vi "AIT 1553 - Create RT Sysdef Tree Messages.vi"(7 "Called From SysDef API (F)":bool, 8 "error in":errorcluster, 9 "RT_Messages":T1[](array[typedef]), 10 "Section Ptr":T3 format="%.0x") -> (0 "error out":errorcluster)   [LabVIEW 2013, in "AIT 1553 Custom Device.lvlib"]
uses:
  AIT 1553 Custom Device.lvlib
  <vilib>/NI Veristand/Custom Device API/Custom Device Item Ref.ctl
  Controls/1553_RT_Message.ctl
  Controls/1553 Param.ctl
  <vilib>/NI Veristand/Custom Device API/Custom Device Channel Type.ctl
  <vilib>/NI Veristand/Custom Device API/Custom Device Channel.ctl
  Controls and Global/Global.vi
  <vilib>/NI Veristand/Custom Device API/Custom Device API.lvlib
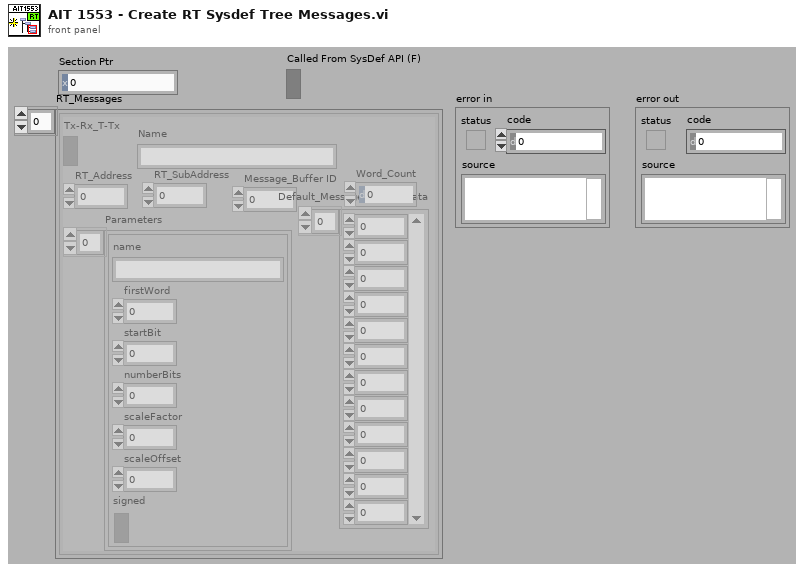
[diagram p1: front panel]
types:
  T1 = typedef "AIT 1553 Custom Device.lvlib/1553_RT_Message.ctl" = cluster{"RT_Address":u8, "RT_SubAddress":u8, "Tx-Rx_T-Tx":bool, "Parameters":T2[], "Message_Buffer ID":u16, "Default_Message_Buffer_Data":u16[], "Word_Count":u8, "Name":string}
  T2 = typedef "AIT 1553 Custom Device.lvlib/1553 Param.ctl" = cluster{"name":string, "firstWord":i32, "startBit":i32, "numberBits":i32, "scaleFactor":dbl, "scaleOffset":dbl, "signed":bool}
  T3 = typedef "Custom Device API.lvlib/Custom Device Item Ref.ctl" = u64
  T4 = typedef "Custom Device API.lvlib/Custom Device Channel Type.ctl" = enum16{"Input", "Output"}
  T5 = typedef "Custom Device API.lvlib/Custom Device Channel.ctl" = cluster{"Type":T4, "Units":string, "Default Value":dbl, "Faultable":bool, "Scalable":bool}
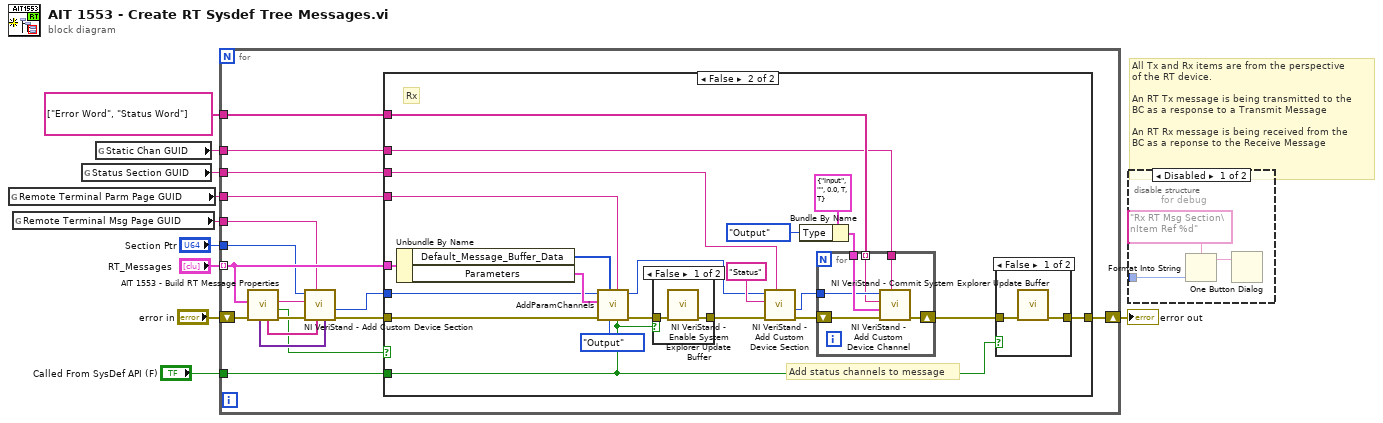
[diagram p0: block diagram]
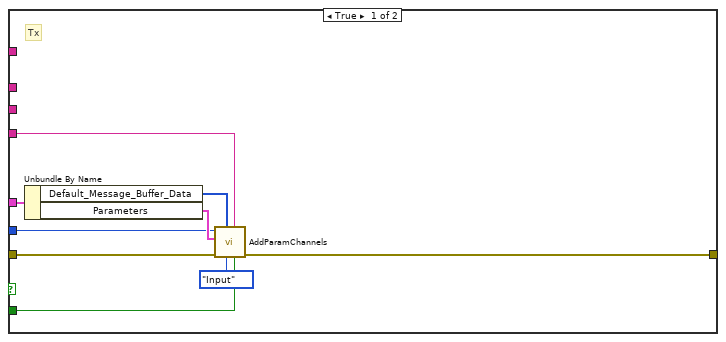
[diagram p3: hidden frame]
diagram:
  # "All Tx and Rx items are from the perspective \nof the RT device.\n\nAn RT Tx message is being transmitted to the \nBC as a response to a Transmit Message\n\nAn RT Rx message is being received from the \nBC as a reponse to the Receive Message"
  n1 = global read "Global.vi" "Remote Terminal Parm Page GUID"() -> (w4:string)
  n2 = global read "Global.vi" "Remote Terminal Msg Page GUID"() -> (w7:string)
  n3 = global read "Global.vi" "Status Section GUID"() -> (w2:string)
  n4 = global read "Global.vi" "Static Chan GUID"() -> (w6:string)
  n5 = for {
    shift-right: [w22] -> w10
    shift-left: "error in" -> [w23]
    tunnel: "Section Ptr" -> [w15]
    tunnel: "RT_Messages" -> [w18] mode=indexing
    tunnel: w7 -> [w17]
    tunnel: w6 -> [w21]
    tunnel: w4 -> [w14]
    tunnel: string[] ["Error Word", "Status Word"] -> [w13]
    tunnel: w2 -> [w12]
    tunnel: "Called From SysDef API (F)" -> [w11]
    n6 = call "AIT 1553 - Build RT Message Properties.vi"("error in (no error)"=w23, "RT_Message"=w18) -> ("error out"=w25:errorcluster, "Tx-Rx  (T=Tx)"=w16:bool, "name"=w24:string, "Prop Names"=w26:string[], "Prop Values"=w27:variant[])  [unwired: 5 in]
    n7 = call <vilib>:"NI VeriStand - Add Custom Device Section.vi"("Property Values"=w27, "Property names"=w26, "GUID (Default Section)"=w17, "error in (no error)"=w25, "Section Name"=w24, "Parent Ref in"=w15) -> ("error out"=w19:errorcluster, "Section Ptr"=w20:T3)  [unwired: 2 in, 2 out]
    n8 = case shown="False" w16 {
      tunnel: w19 -> [w35 w57]
      tunnel: w20 -> [w34 w53]
      tunnel: [w29 w39] -> w22
      tunnel: w21 -> [_ w44]
      tunnel: w18 -> [w32 w55]
      tunnel: w14 -> [w30 w52]
      tunnel: w13 -> [_ w45]
      tunnel: w12 -> [_ w43]
      tunnel: w11 -> [w28 w38]
      frame True {
        # "Tx"
        n9 = Unbundle By Name(w32) -> ("Default_Message_Buffer_Data"=w31:u16[], "Parameters"=w36:T2[])
        n10 = call "AddParamChannels.vi"("Called From SysDef API (F)"=w28, "Parm Page GUID"=w30, "Type"=Custom_Device_Channel_Type."Input", "Default Message Data"=w31, "error in"=w35, "Parameters to add"=w36, "Node Ref In"=w34) -> ("error out"=w29:errorcluster)  [unwired: 3 in, 1 out]
      }
      frame False {
        # "Add status channels to message"
        # "Rx"
        n11 = Unbundle By Name(w55) -> ("Default_Message_Buffer_Data"=w54:u16[], "Parameters"=w58:T2[])
        n12 = call "AddParamChannels.vi"("Called From SysDef API (F)"=w38, "Parm Page GUID"=w52, "Type"=Custom_Device_Channel_Type."Output", "Default Message Data"=w54, "error in"=w57, "Parameters to add"=w58, "Node Ref In"=w53) -> ("error out"=w41:errorcluster, "Node Ref Out"=w42:T3)  [unwired: 3 in]
        n13 = case shown="False" w38 {
          tunnel: w41 -> [w63 w64]
          tunnel: [w62 w64] -> w40
          frame False {
            n14 = call <vilib>:"NI VeriStand - Enable System Explorer Update Buffer.vi"("error in (no error)"=w63) -> ("error out"=w62:errorcluster)  [unwired: 10 in]
          }
          frame True {
          }
        }
        n15 = call <vilib>:"NI VeriStand - Add Custom Device Section.vi"("GUID (Default Section)"=w43, "error in (no error)"=w40, "Section Name"="Status", "Parent Ref in"=w42) -> ("error out"=w49:errorcluster, "Section Ptr"=w50:T3)  [unwired: 4 in, 2 out]
        n16 = Bundle By Name(cluster=T5 {"Type"=enum."Input", "Units"="", "Default Value"=0.0, "Faultable"=TRUE, "Scalable"=TRUE} ("Channel"), "Type"=Custom_Device_Channel_Type."Output") -> (w48:T5)
        n17 = for {
          tunnel: w48 -> [w69]
          tunnel: w44 -> [w68]
          tunnel: w50 -> [w66]
          tunnel: w45 -> [w65] mode=indexing
          shift-right: [w70] -> w37
          shift-left: w49 -> [w67]
          n18 = call <vilib>:"NI VeriStand - Add Custom Device Channel.vi"("GUID (Default Channel)"=w68, "error in (no error)"=w67, "Channel"=w69, "Channel Name"=w65, "Parent Ref in"=w66) -> ("error out"=w70:errorcluster)  [unwired: 3 in, 3 out]
        }
        n19 = case shown="False" w38 {
          tunnel: w37 -> [w60 w61]
          tunnel: [w59 w61] -> w39
          frame False {
            n20 = call <vilib>:"NI VeriStand - Commit System Explorer Update Buffer.vi"("error in (no error)"=w60) -> ("error out"=w59:errorcluster)  [unwired: 10 in]
          }
          frame True {
          }
        }
      }
    }
  }
  "error out" <- w10
  n21 = disable-structure shown="Disabled" {
    disable-tunnel: _ -> [w71 _]
    frame Disabled {
      # "for debug"
      n22 = Format Into String(format string="Rx RT Msg Section\nItem Ref %d" ("message"), w71) -> (resulting string=w73:string)  [unwired: 2 in, 1 out]
      n23 = One Button Dialog(message=w73) -> ()  [unwired: 1 in, 1 out]
    }
    frame Enabled {
    }
  }
